vi "setUp.vi"(8 "error in (no error)":errorcluster, 11 "reference in":refnum<class "Single Consumer Test Case.lvclass">) -> (0 "error out":errorcluster, 3 "reference out":refnum<class "Single Consumer Test Case.lvclass">)   [LabVIEW 2017, in "Single Consumer Test Case.lvclass"]
doc: "setUp runs prior to the test method during test execution. Use this method to initialize any object data required by your tests."
uses:
  Single Consumer Test Case.lvclass
  C:/Program Files (x86)/National Instruments/LabVIEW 2017/vi.lib/addons/_JKI Toolkits/VI Tester/TestCase.llb/TestCase.lvclass
  Producer/Abstract Producer/Abstract Producer.lvclass
  Parameters/Abstract Init Parameters/Abstract Init Parameters.lvclass
  Message Queue/Message Queue/Message Queue.lvclass
  C:/github/niveristand-custom-device-message-library/Source/Message Queue/Abstract Message Queue/Abstract Message Queue.lvclass
  Support/Consumers/Test Consumer/Test Consumer.lvclass
  C:/github/niveristand-custom-device-message-library/Source/Consumer/Abstract Consumer/Abstract Consumer.lvclass
  Support/Message String Action.ctl
  Support/Message List Action.ctl
  Single Consumer Test Case.lvclass/Single Consumer Test Case.ctl
  <vilib>/addons/_JKI Toolkits/VI Tester/TestCase.llb/TestCase.lvclass
  Consumer/Abstract Consumer/Abstract Consumer.lvclass
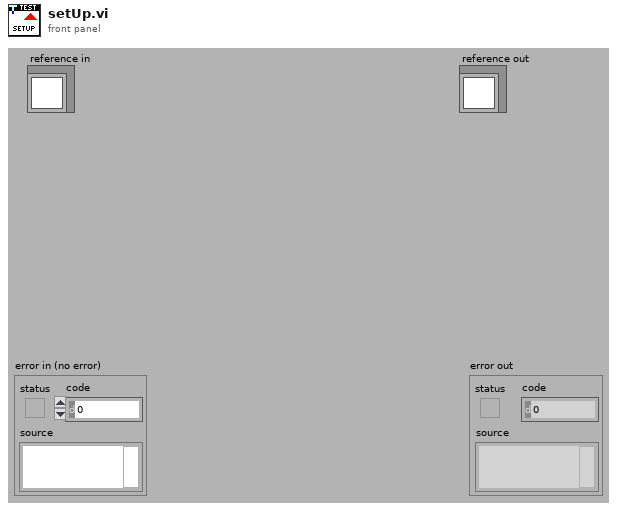
[diagram p1: front panel]
types:
  T1 = typedef "Message List Action.ctl" = enum16{"Get", "Add", "Reset"}
  T2 = typedef "Message String Action.ctl" = enum16{"Get String", "Set String", "Reset"}
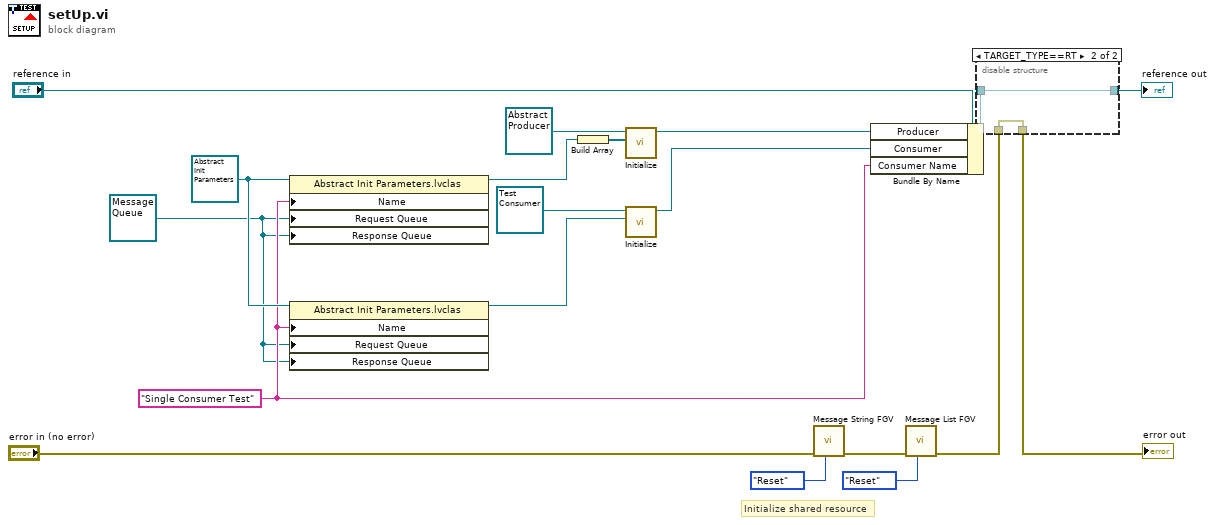
[diagram p0: block diagram]
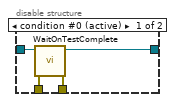
[diagram p2: hidden frame]
diagram:
  w7 = refnum<class "Message Queue.lvclass"> refnum ("Messaging.lvlib:Message Queue.lvlib:Message Queue.lvclass")
  w8 = "Single Consumer Test" ("Name")
  w15 = refnum<class "Abstract Init Parameters.lvclass"> refnum ("Message Queue Library.lvlib:Abstract Init Parameters.lvclass")
  # "Initialize shared resource"
  n1 = property class="Abstract Init Parameters.lvclas"(reference=w15, "Name"=w8, "Request Queue"=w7, "Response Queue"=w7) -> (reference out=w12:refnum<class "Abstract Init Parameters.lvclass">)  [unwired: 1 in, 1 out]
  n2 = property class="Abstract Init Parameters.lvclas"(reference=w15, "Name"=w8, "Request Queue"=w7, "Response Queue"=w7) -> (reference out=w11:refnum<class "Abstract Init Parameters.lvclass">)  [unwired: 1 in, 1 out]
  n3 = Build Array(w12) -> (w13:refnum<class "Abstract Init Parameters.lvclass">[])
  n4 = call "Initialize.vi"("Parameters in"=w13, "Abstract Producer in"=refnum<class "Abstract Producer.lvclass"> refnum ("Messaging.lvlib:Producer.lvlib:Abstract Producer.lvclass")) -> ("Abstract Producer out"=w10:refnum<class "Abstract Producer.lvclass">)  [unwired: 8 in, 1 out]
  n5 = call "Initialize.vi"("Parameters in"=w11, "Abstract Consumer in"=refnum<class "Test Consumer.lvclass"> refnum ("Test Consumer.lvclass")) -> ("Abstract Consumer out"=w9:refnum<class "Test Consumer.lvclass">)  [unwired: 8 in, 1 out]
  n6 = call "Message String FGV.vi"("Action"=Message_String_Action."Reset", "error in (no error)"="error in (no error)") -> ("error out"=w5:errorcluster)  [unwired: 8 in, 1 out]
  n7 = Bundle By Name(cluster="reference in", "Producer"=w10, "Consumer"=w9, "Consumer Name"=w8) -> (w16:refnum<class "Single Consumer Test Case.lvclass">)
  n8 = call "Message List FGV.vi"("Action (Get)"=Message_List_Action."Reset", "error in (no error)"=w5) -> ("error out"=w4:errorcluster)  [unwired: 8 in, 1 out]
  n9 = disable-structure shown="TARGET_TYPE==RT" {
    disable-tunnel: w4 -> [w23 w24]
    disable-tunnel: [w22 w24] -> w19
    disable-tunnel: [w21 w25] -> w18
    disable-tunnel: w16 -> [w20 w25]
    frame condition #0 (active) {
      n10 = call <vilib>:"WaitOnTestComplete.vi"("error in (no error)"=w23, "TestCase in"=w20) -> ("error out"=w22:errorcluster, "TestCase out"=w21:refnum<class "Single Consumer Test Case.lvclass">)  [unwired: 8 in]
    }
    frame condition #1 {
    }
  }
  "error out" <- w19
  "reference out" <- w18
